vi "Jet in scan on or off.vi"(8 "error in (no error)":errorcluster, 10 "Jet On Times":T1 {"gas jet on time" format="%#_6p"}, 11 "GasJetOn":bool) -> (0 "error out":errorcluster)   [LabVIEW 2020]
uses:
  Jet on times.ctl
panel:
  out "Array":string[](array[string])
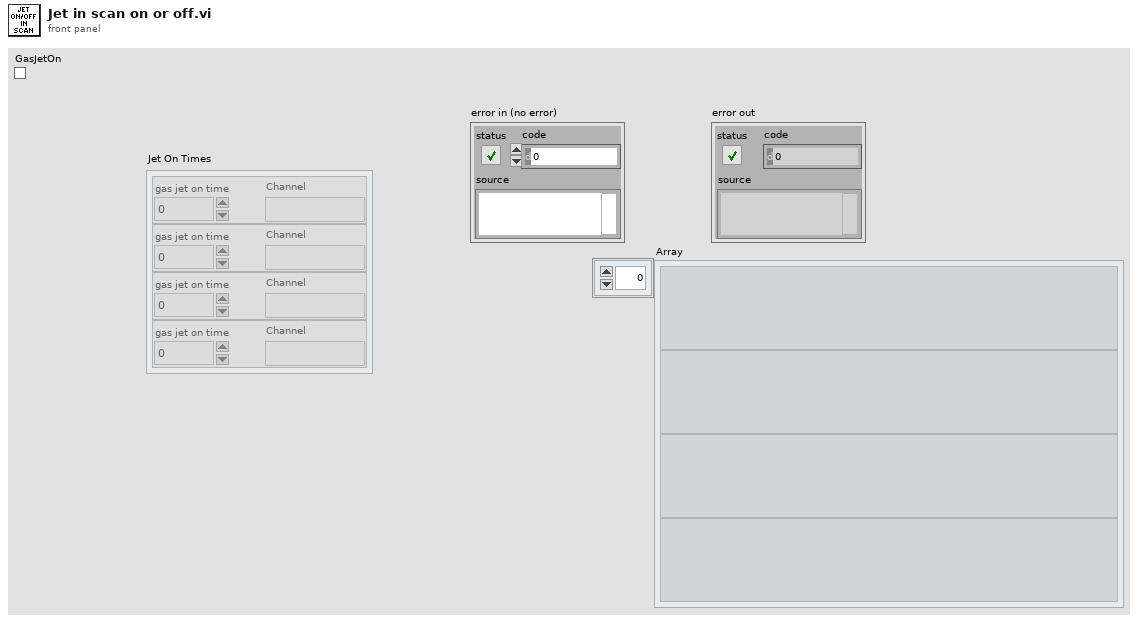
[diagram p1: front panel]
types:
  T1 = typedef "Jet on times.ctl" = cluster{"gas jet on time":dbl, "Channel":string}[]
  T2 = typedef "mysql_authentication.ctl" = cluster{"User":string, "Password":string, "Database":string}
  T3 = cluster{"Port":u16, "IP Address":string, "Authentication":T2}
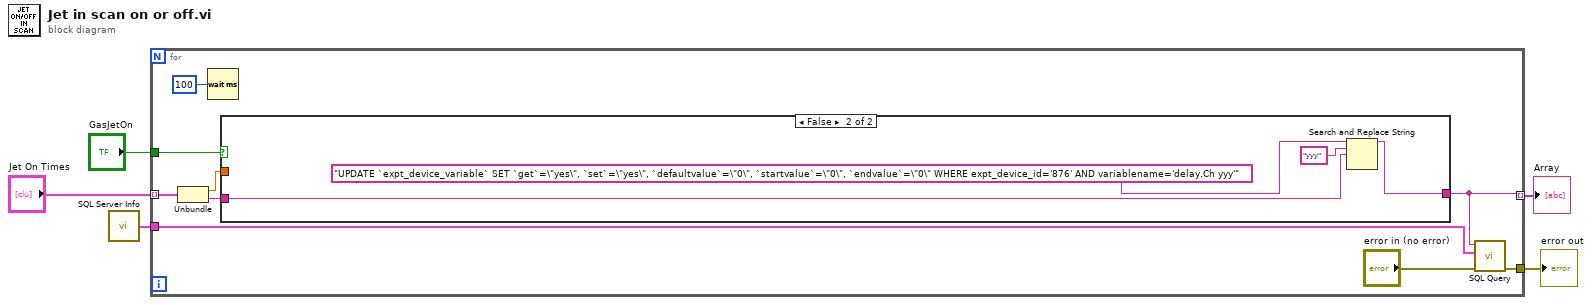
[diagram p0: block diagram]
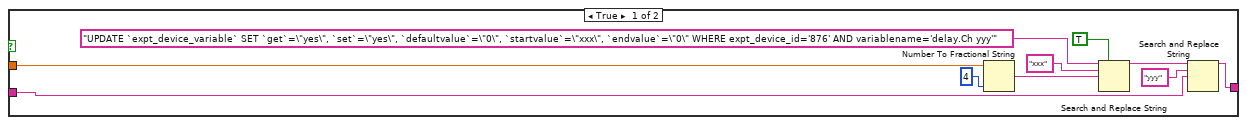
[diagram p2: hidden frame]
diagram:
  n1 = call "SQL Server Info.vi"() -> ("SQL Server Info"=w2:T3)
  n2 = for {
    tunnel: "GasJetOn" -> [w14]
    tunnel: "Jet On Times" -> [w9] mode=indexing
    tunnel: [w12] -> w3
    tunnel: w2 -> [w11]
    tunnel: [w6] -> w1 mode=indexing
    n3 = Unbundle(w9) -> ("gas jet on time"=w8:dbl, "Channel"=w7:string)
    n4 = Wait (ms)(milliseconds to wait=u32 100) -> ()  [unwired: 1 out]
    n5 = case shown="False" w14 {
      tunnel: [w18 w26] -> w6
      tunnel: w8 -> [w16 _]
      tunnel: w7 -> [w15 w25]
      frame True {
        n6 = Number To Fractional String(number=w16, precision (6)=i16 4) -> (F-format string=w21:string)  [unwired: 2 in]
        n7 = Search and Replace String(replace all?=TRUE ("replace all? (F)"), input string="UPDATE `expt_device_variable` SET `get`=\"yes\", `set`=\"yes\", `defaultvalue`=\"0\", `startvalue`=\"xxx\", `endvalue`=\"0\" WHERE expt_device_id='876' AND variablename='delay.Ch yyy'" ("Query"), search string="xxx", replace string=w21) -> (result string=w19:string)  [unwired: 4 in, 3 out]
        n8 = Search and Replace String(input string=w19, search string="yyy", replace string=w15) -> (result string=w18:string)  [unwired: 5 in, 3 out]
      }
      frame False {
        n9 = Search and Replace String(input string="UPDATE `expt_device_variable` SET `get`=\"yes\", `set`=\"yes\", `defaultvalue`=\"0\", `startvalue`=\"0\", `endvalue`=\"0\" WHERE expt_device_id='876' AND variablename='delay.Ch yyy'" ("Query"), search string="yyy", replace string=w25) -> (result string=w26:string)  [unwired: 5 in, 3 out]
      }
    }
    n10 = call "SQL Query.vi"("error in (no error)"="error in (no error)", "SQL Server Info"=w11, "Query"=w6) -> ("error out"=w12:errorcluster)  [unwired: 7 in, 1 out]
  }
  "error out" <- w3
  "Array" <- w1
